vi "Ramp_Linear.vi"(0 "Acquisition Rate (20000) / Hz":dbl=20000.0, 9 "Ramp Time (1) /s":dbl=1.0, 11 "Error in":errorcluster, 12 "Ramp Height (10) / nm":dbl=10.0, 13 "DC Bias (0.2) / V":dbl=0.2) -> (4 "Piezo Ramp Out / nm":dbl[](array[numeric]), 8 "Bias Ramp Out / V":dbl[](array[numeric]), 15 "Error Out":errorcluster)   [LabVIEW 2023]
uses:
  <vilib>/Analysis/NI_AALBase.lvlib
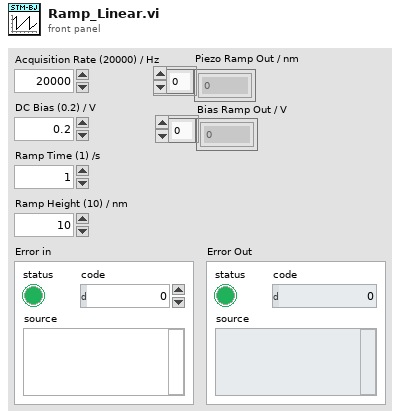
[diagram p1: front panel]
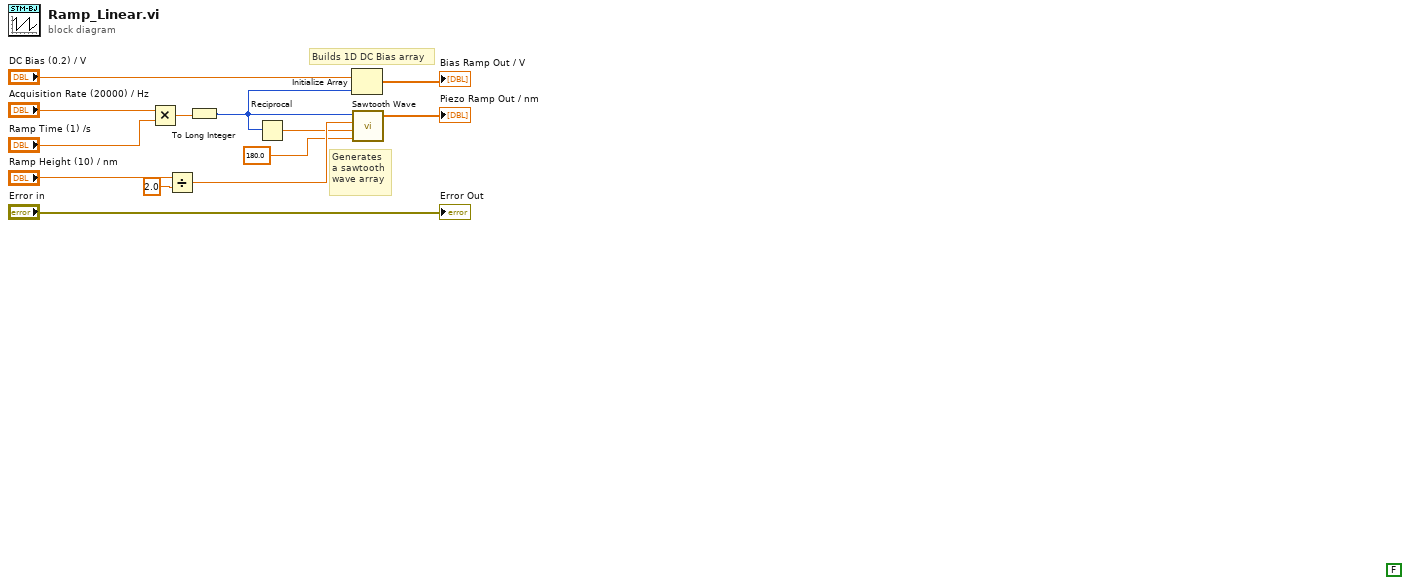
[diagram p0: block diagram]
diagram:
  (unwired) FALSE
  # "Generates\na sawtooth\nwave array"
  # "Builds 1D DC Bias array"
  n1 = Multiply(x="Acquisition Rate (20000) / Hz", y="Ramp Time (1) /s") -> (x*y=w6:dbl)
  n2 = Divide(x="Ramp Height (10) / nm", y=2.0) -> (x/y=w10:dbl)
  n3 = To Long Integer(number=w6) -> (32bit integer=w5:i32)
  n4 = Reciprocal(x=w5) -> (1/x=w7:dbl)
  n5 = Initialize Array("DC Bias (0.2) / V", w5) -> (→"Bias Ramp Out / V":dbl[])
  n6 = call <vilib>:"Sawtooth Wave.vi"("samples"=w5, "amplitude"=w10, "frequency"=w7, "phase in"=180.0) -> ("sawtooth wave"=→"Piezo Ramp Out / nm":dbl[])  [unwired: 1 in, 2 out]
  "Error Out" <- "Error in"
